vi "test median filter.vi"() -> ()   [LabVIEW 2016]
uses:
  <vilib>/gmath/NI_Gmath.lvlib
panel:
  out "Array":dbl[](array[numeric])
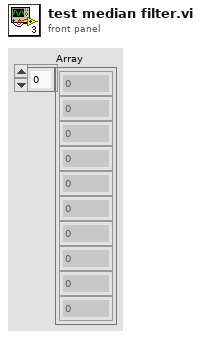
[diagram p1: front panel]
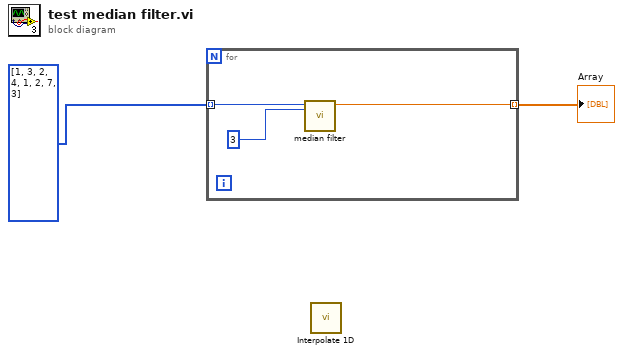
[diagram p0: block diagram]
diagram:
  n1 = for {
    tunnel: i32[] [1, 3, 2, 4, 1, 2, 7, 3] -> [w5] mode=indexing
    tunnel: [w3] -> w1 mode=indexing
    n2 = call "median filter.vi"("Sample Length"=3, "Element Input"=w5) -> ("Output Element"=w3:dbl)  [unwired: 9 in]
  }
  "Array" <- w1
  n3 = call <vilib>:"Interpolate 1D.vi"() -> ()  [unwired: 9 in, 3 out]
